vi "Dycometal CCK-25.vi"() -> ()   [LabVIEW 2017]
uses:
  <vilib>/Utility/file.llb/Write Delimited Spreadsheet (DBL).vi
panel:
  out "Frecuencia Fijada":i32=20
  out "Out 1.1":refnum<visa-resource-name>
  out "Out 1.2":errorcluster
  out "Out 2.1":refnum<visa-resource-name>
  out "Out 2.2":errorcluster
  out "Tab Control":enum32{"Comunicación", "Parámetros", "Medición"}(tab)
  in  "Parámetros 1":bool
  in  "Configuración COM - C. Climática":T1={"Velocidad de transmisión"=9600, "Paridad"=0, "Bits de parada"=10} caption="Configuración COM" {"Bits de parada" items=["0"=10, "1,5"=15, "2"=20]; "Paridad" items=["No", "Impar", "Par", "Marcada", "Espaciada"]; "Velocidad de transmisión" items=["300"=300, "600"=600, "1200"=1200, "2400"=2400, "4800"=4800, "9600"=9600]}
  in  "Parámetro prioritario:":bool=TRUE
  in  "Puerto COM - C. Climática":refnum<visa-resource-name> caption="Puerto COM"
  in  "Puerto COM - Medidor LCR":refnum<visa-resource-name> caption="Puerto COM"
  in  "Configuración COM - Medidor LCR":T2={"Velocidad de transmisión"=9600, "Paridad"=0, "Bits de datos"=7, "Bits de parada"=10, "Control flujo de datos"=0} caption="Configuración COM" {"Bits de parada" items=["1"=10, "1,5"=15, "2"=20]; "Bits de datos" items=["7"=7, "8"=8]; "Paridad" items=["No", "Impar", "Par", "Marcada", "Espaciada"]; "Control flujo de datos" items=["No", "XON/XOFF", "RTS/CTS", "XON/XOFF & RTS/CTS", "DTR/DSR", "XON/XOFF & DTR/DSR"]; "Velocidad de transmisión" items=["300"=300, "600"=600, "1200"=1200, "2400"=2400, "4800"=4800, "9600"=9600]}
  in  "Medición 1":bool
  in  "Frecuencia Final":i32(ring)=68 items=["20 Hz", "24 Hz", "25 Hz", "30 Hz", "36 Hz", "40 Hz", "45 Hz", "50 Hz", "60 Hz", "72 Hz", "75 Hz", "80 Hz", "90 Hz", "100 Hz", "120 Hz", "150 Hz", "180 Hz", "200 Hz", "240 Hz", "250 Hz", "300 Hz", "360 Hz", "400 Hz", "450 Hz", "500 Hz", "600 Hz", "720 Hz", "750 Hz", "800 Hz", "900 Hz", "1k Hz", "1,2k Hz", "1,5k Hz", "1,8k Hz", "2k Hz", "2,4k Hz", "2,5k Hz", "3k Hz", "3,6k Hz", "4k Hz", "4,5k Hz", "5k Hz", "6k Hz", "7,2k Hz", "7,5k Hz", "8k Hz", "9k Hz", "10k Hz", "12k Hz", "15k Hz", "18k Hz", "20k Hz", "24k Hz", "25k Hz", "30k Hz", "36k Hz", "40k Hz", "45k Hz", "50k Hz", "60k Hz", "72k Hz", "75k Hz", "80k Hz", "90k Hz", "100k Hz", "120k Hz", "150k Hz", "180k Hz", "200k Hz"]
  in  "Tipo de Circuito":u16(ring)=2 items=["Serie", "Paralelo", "Auto"]
  in  "Formato de Salida":u16(ring) items=["Auto", "L+Q", "L+R", "C+D", "C+R", "R+Q", "Z+Theta", "Y+Theta", "R+X", "G+B", "N+Theta", "M"]
  in  "Escala Manual":u8(ring)=1 items=["Escala 1: 3 Ohms"=1, "Escala 2: 100 Ohms"=2, "Escala 3: 1,6 kOhms"=3, "Escala 4: 25 kOhms"=4, "Escala 5: 500 kOhms"=5, "Escala 6: 100 MOhms"=6]
  in  "Modo Autoescala":bool=TRUE
  in  "Frecuencia Inicial":i32(ring) items=["20 Hz", "24 Hz", "25 Hz", "30 Hz", "36 Hz", "40 Hz", "45 Hz", "50 Hz", "60 Hz", "72 Hz", "75 Hz", "80 Hz", "90 Hz", "100 Hz", "120 Hz", "150 Hz", "180 Hz", "200 Hz", "240 Hz", "250 Hz", "300 Hz", "360 Hz", "400 Hz", "450 Hz", "500 Hz", "600 Hz", "720 Hz", "750 Hz", "800 Hz", "900 Hz", "1k Hz", "1,2k Hz", "1,5k Hz", "1,8k Hz", "2k Hz", "2,4k Hz", "2,5k Hz", "3k Hz", "3,6k Hz", "4k Hz", "4,5k Hz", "5k Hz", "6k Hz", "7,2k Hz", "7,5k Hz", "8k Hz", "9k Hz", "10k Hz", "12k Hz", "15k Hz", "18k Hz", "20k Hz", "24k Hz", "25k Hz", "30k Hz", "36k Hz", "40k Hz", "45k Hz", "50k Hz", "60k Hz", "72k Hz", "75k Hz", "80k Hz", "90k Hz", "100k Hz", "120k Hz", "150k Hz", "180k Hz", "200k Hz"]
  in  "Bol_Escalado_Hum":bool=TRUE
  in  "Bol_Escalado_Temp":bool=TRUE
  in  "Escalado Temp":sgl caption="Escalado" min=0 max=100 step=5
  in  "Error Temp":sgl caption="Error" min=0 max=100
  in  "Error Hum":sgl caption="Error" min=0 max=100
  in  "Escalado Hum":sgl caption="Escalado" min=0 max=100 step=5
  in  "Hum Final":sgl=10.0 caption="Final" min=10 max=98 step=5
  in  "Temp Final":sgl caption="Final" min=0 max=100 step=5
  in  "Temperatura Inicial":sgl caption="Inicio" min=0 max=100 step=5
  in  "Humedad Inicial":sgl=10.0 caption="Inicio" min=10 max=98 step=5
  in  "Ruta a excel de almacenaje":path
  in  "Regimen Permanente":dbl min=0.0 step=900.0 format="%<%H:%M>t"
  in  "Iniciar":bool
  in  "Parámetros 2":bool
  out "Gráfica":T3(graph)={"Temperatura Medida"=20.209763, "Humedad Medida"=41.667168}
  out "Humedad Fijada":sgl
  out "Temperatura Fijada":sgl
  out "En regimen permanente:":dbl format="%<%H:%M>t"
  in  "Obtener datos de gráfica":bool
  out "Últimas mediciones":dbl[][](array[numeric]) format="%^#_4e"
  in  "Parar":bool
  # "Cámara Climática"
  # "Medidor LCR"
  # "Cámara Climática"
  # "Medidor LCR"
  # "¿Bucle en Temperatura o Humedad?"
  # "Última Medición"
  # "Temperatura"
  # "Humedad"
  # "Frecuencia"
  # "Parámetro 1"
  # "Parámetro 2"
  # "Temperatura Medida"
  # "Humedad Medida"
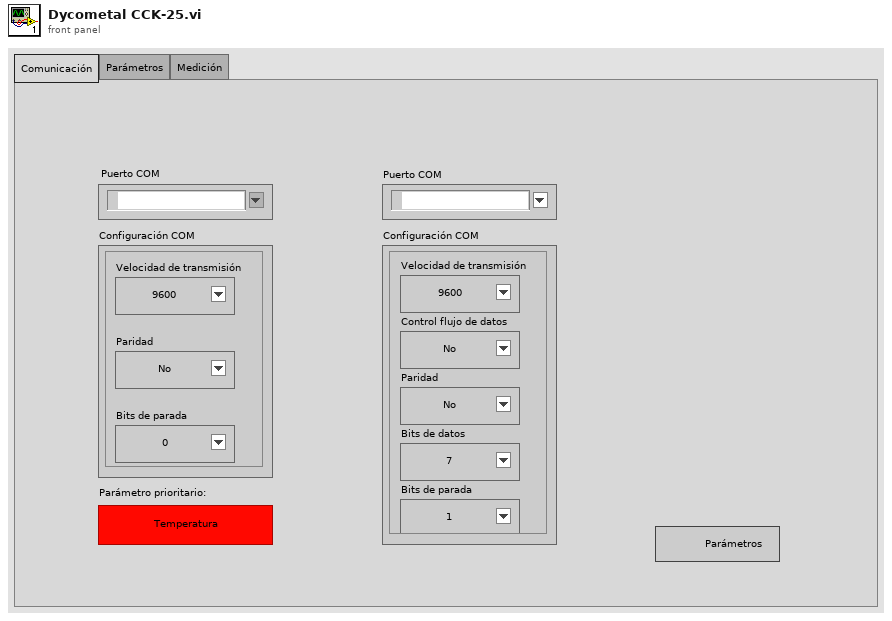
[diagram p1: front panel]
types:
  T1 = cluster{"Velocidad de transmisión":u32, "Paridad":u16, "Bits de parada":u16}
  T2 = cluster{"Velocidad de transmisión":u32, "Paridad":u16, "Bits de datos":u16, "Bits de parada":u16, "Control flujo de datos":u16}
  T3 = cluster{"Temperatura Medida":sgl, "Humedad Medida":sgl}
  T4 = enum8{"Enabled", "Disabled", "Disabled and Grayed Out"}
  T5 = cluster{"Temperatura Medida":sgl, "Humedad Medida":sgl}[]
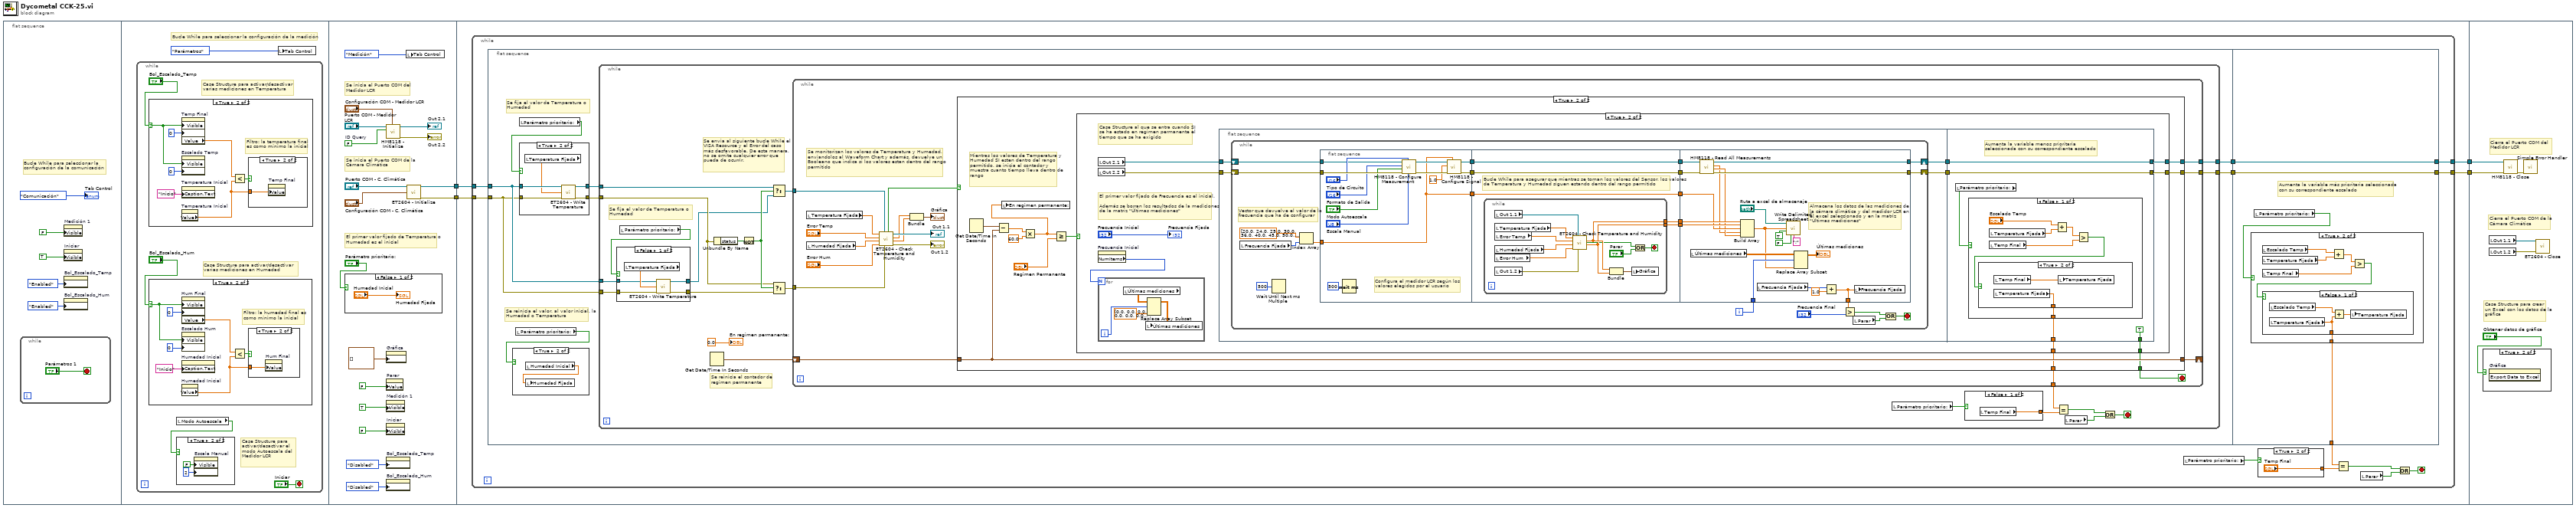
[diagram p0: block diagram]
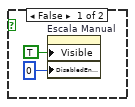
[diagram p2: hidden frame]
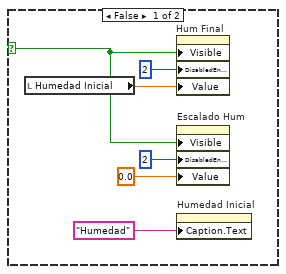
[diagram p3: hidden frame]
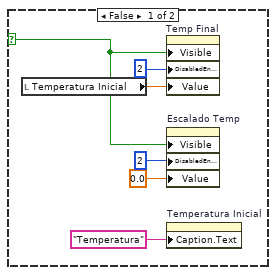
[diagram p5: hidden frame]
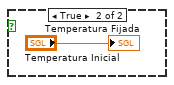
[diagram p7: hidden frame]
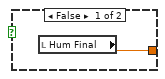
[diagram p8: hidden frame]
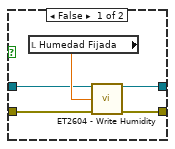
[diagram p9: hidden frame]
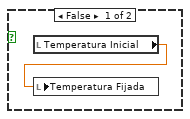
[diagram p10: hidden frame]
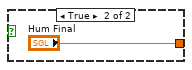
[diagram p11: hidden frame]
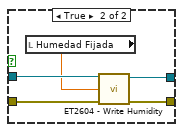
[diagram p12: hidden frame]
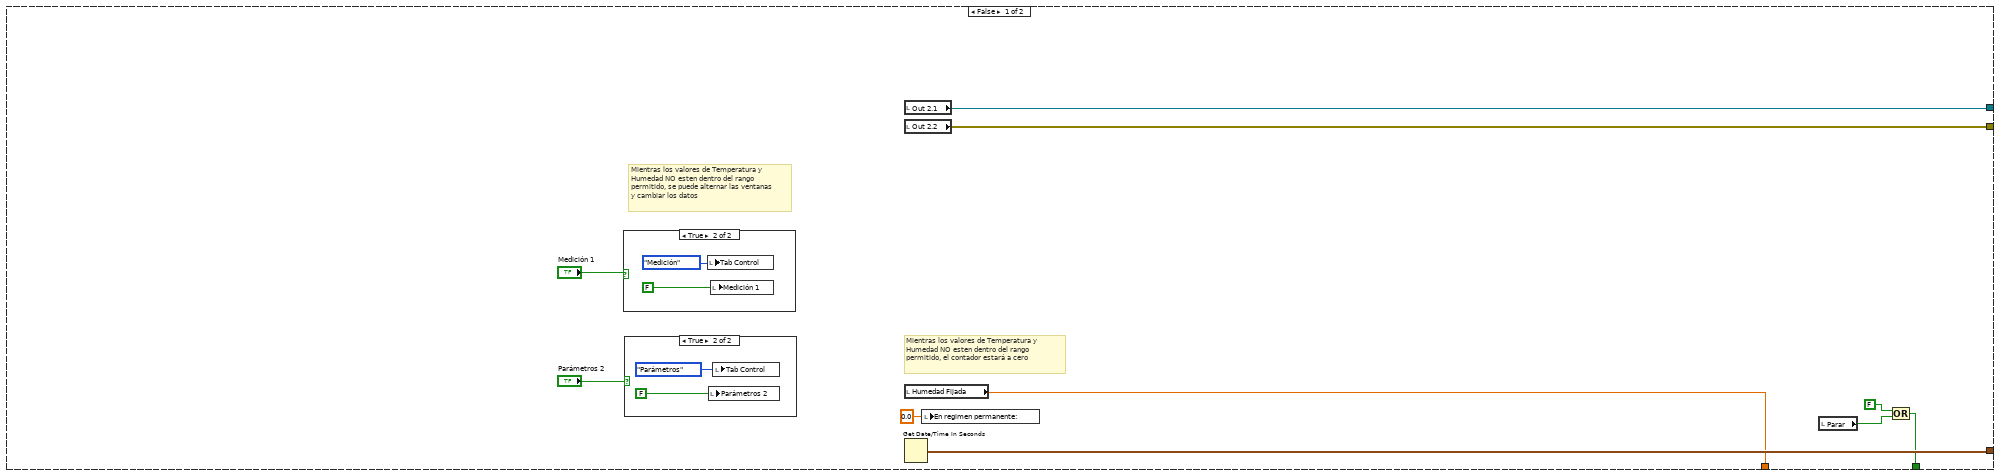
[diagram p13: hidden frame]
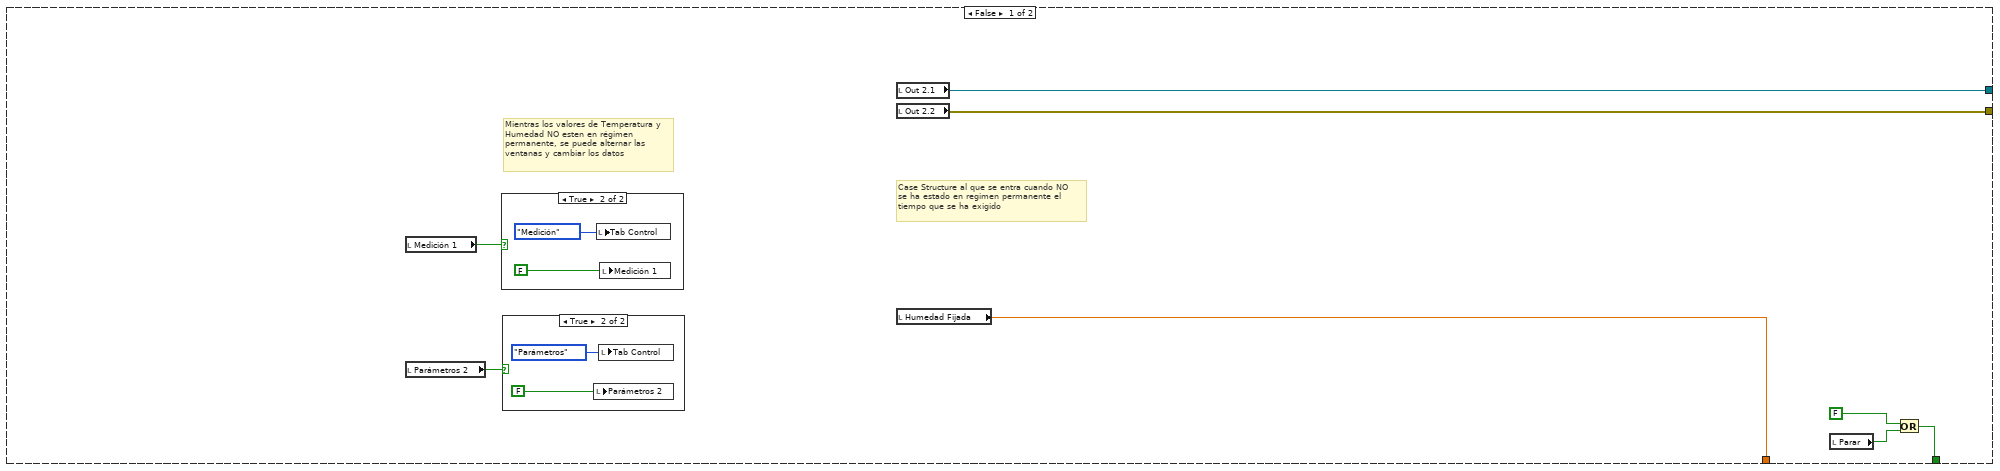
[diagram p16: hidden frame]
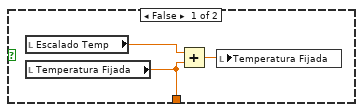
[diagram p19: hidden frame]
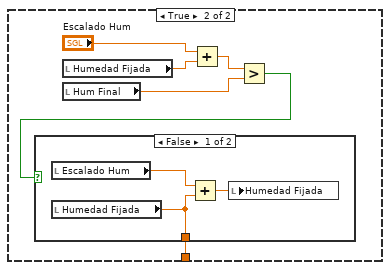
[diagram p20: hidden frame]
diagram:
  n1 = flat-sequence {
    tunnel: [w51] -> w4
    tunnel: [w50] -> w3
    tunnel: w4 -> [w68]
    tunnel: w3 -> [w67]
    tunnel: [w70] -> w2
    tunnel: [w69] -> w1
    tunnel: w2 -> [w339]
    tunnel: w1 -> [w340]
    frame #0 {
      # "Bucle While para seleccionar la configuración de la comunicación"
      n2 = while {
        stop <- "Parámetros 1" stop-if-true
      }
      n3 = property on="Medición 1" class="Bool (strict)"("Visible"=FALSE) -> ()  [unwired: 2 in, 2 out]
      n4 = property on="Iniciar" class="Bool"("Visible"=TRUE) -> ()  [unwired: 2 in, 2 out]
      n5 = property on="Bol_Escalado_Temp" class="Bool (strict)"("DisabledEnum"=T4."Enabled" ("Disabled")) -> ()  [unwired: 2 in, 2 out]
      n6 = property on="Bol_Escalado_Hum" class="Bool (strict)"("DisabledEnum"=T4."Enabled" ("Disabled")) -> ()  [unwired: 2 in, 2 out]
      "Tab Control" <- enum32{"Comunicación", "Parámetros", "Medición"}."Comunicación" ("Tab Control")
    }
    frame #1 {
      # "Bucle While para seleccionar la configuración de la medición"
      n7 = while {
        stop <- "Iniciar" stop-if-true
        # "Case Structure para activar/desactivar el modo Autoescala del Medidor LCR"
        # "Case Structure para activar/desactivar varias mediciones en Humedad"
        # "Case Structure para activar/desactivar varias mediciones en Temperatura"
        n8 = case shown="True" "Bol_Escalado_Temp" {
          selector: "Bol_Escalado_Temp" -> [w39 w46]
          frame False {
            n9 = local read "Temperatura Inicial"() -> (w35:sgl)
            n10 = property on="Temp Final" class="DigNum (strict)"("Visible"=w39, "DisabledEnum"=u8 2, "Value"=w35) -> ()  [unwired: 2 in, 2 out]
            n11 = property on="Escalado Temp" class="DigNum (strict)"("Visible"=w39, "DisabledEnum"=u8 2, "Value"=sgl 0.0 ("Humedad Escalado")) -> ()  [unwired: 2 in, 2 out]
            n12 = property on="Temperatura Inicial" class="DigNum (strict)"("Caption.Text"="Temperatura") -> ()  [unwired: 2 in, 2 out]
          }
          frame True {
            # "Filtro: la temperatura final es como mínimo la inicial"
            n13 = property on="Temp Final" class="DigNum (strict)"("Visible"=w46, "DisabledEnum"=u8 0) -> ("Value"=w42:sgl)  [unwired: 2 in, 2 out]
            n14 = property on="Escalado Temp" class="DigNum (strict)"("Visible"=w46, "DisabledEnum"=u8 0) -> ()  [unwired: 2 in, 2 out]
            n15 = property on="Temperatura Inicial" class="DigNum (strict)"("Caption.Text"="Inicio") -> ()  [unwired: 2 in, 2 out]
            n16 = property on="Temperatura Inicial" class="DigNum (strict)"() -> ("Value"=w40:sgl)  [unwired: 2 in, 2 out]
            n17 = Less?(x=w42, y=w40) -> (x < y?=w41:bool)
            n18 = case shown="True" w41 {
              tunnel: w40 -> [_ w47]
              frame False {
              }
              frame True {
                n19 = property on="Temp Final" class="DigNum (strict)"("Value"=w47) -> ()  [unwired: 2 in, 2 out]
              }
            }
          }
        }
        n20 = case shown="True" "Bol_Escalado_Hum" {
          selector: "Bol_Escalado_Hum" -> [w25 w32]
          frame False {
            n21 = local read "Humedad Inicial"() -> (w21:sgl)
            n22 = property on="Hum Final" class="DigNum (strict)"("Visible"=w25, "DisabledEnum"=u8 2, "Value"=w21) -> ()  [unwired: 2 in, 2 out]
            n23 = property on="Escalado Hum" class="DigNum (strict)"("Visible"=w25, "DisabledEnum"=u8 2, "Value"=sgl 0.0 ("Humedad Escalado")) -> ()  [unwired: 2 in, 2 out]
            n24 = property on="Humedad Inicial" class="DigNum (strict)"("Caption.Text"="Humedad") -> ()  [unwired: 2 in, 2 out]
          }
          frame True {
            # "Filtro: la humedad final es como mínimo la inicial"
            n25 = property on="Hum Final" class="DigNum (strict)"("Visible"=w32, "DisabledEnum"=u8 0) -> ("Value"=w28:sgl)  [unwired: 2 in, 2 out]
            n26 = property on="Escalado Hum" class="DigNum (strict)"("Visible"=w32, "DisabledEnum"=u8 0) -> ()  [unwired: 2 in, 2 out]
            n27 = property on="Humedad Inicial" class="DigNum (strict)"("Caption.Text"="Inicio") -> ()  [unwired: 2 in, 2 out]
            n28 = property on="Humedad Inicial" class="DigNum (strict)"() -> ("Value"=w27:sgl)  [unwired: 2 in, 2 out]
            n29 = Less?(x=w28, y=w27) -> (x < y?=w26:bool)
            n30 = case shown="True" w26 {
              tunnel: w27 -> [_ w33]
              frame False {
              }
              frame True {
                n31 = property on="Hum Final" class="DigNum (strict)"("Value"=w33) -> ()  [unwired: 2 in, 2 out]
              }
            }
          }
        }
        n32 = local read "Modo Autoescala"() -> (w12:bool)
        n33 = case shown="True" w12 {
          frame False {
            n34 = property on="Escala Manual" class="Ring (strict)"("Visible"=TRUE, "DisabledEnum"=u8 0) -> ()  [unwired: 2 in, 2 out]
          }
          frame True {
            n35 = property on="Escala Manual" class="Ring (strict)"("Visible"=FALSE, "DisabledEnum"=u8 2) -> ()  [unwired: 2 in, 2 out]
          }
        }
      }
      n36 = local write "Tab Control"(enum32{"Comunicación", "Parámetros", "Medición"}."Parámetros" ("Tab Control")) -> ()
    }
    frame #2 {
      w52 = FALSE  # ID Query
      # "El primer valor fijado de Temperatura o Humedad es el inicial"
      # "Se inicia el Puerto COM de la Cámara Climática"
      # "Se inicia el Puerto COM del Medidor LCR"
      n37 = case shown="False" "Parámetro prioritario:" {
        frame False {
          "Humedad Fijada" <- "Humedad Inicial"
        }
        frame True {
          "Temperatura Fijada" <- "Temperatura Inicial"
        }
      }
      n38 = call "HM8118 - Initialize.vi"("Serial Configuration"="Configuración COM - Medidor LCR", "ID Query (True)"=w52, "VISA resource name"="Puerto COM - Medidor LCR") -> ("error out"=→"Out 2.2":errorcluster, "VISA resource name out"=→"Out 2.1":refnum<visa-resource-name>)  [unwired: 7 in]
      n39 = property on="Gráfica" class="WFChart (strict)"("History Data"=T5 []) -> ()  [unwired: 2 in, 2 out]
      n40 = property on="Parar" class="Bool (strict)"("Value"=FALSE ("Cancel Button")) -> ()  [unwired: 2 in, 2 out]
      n41 = property on="Medición 1" class="Bool (strict)"("Visible"=TRUE) -> ()  [unwired: 2 in, 2 out]
      n42 = property on="Iniciar" class="Bool"("Visible"=FALSE) -> ()  [unwired: 2 in, 2 out]
      n43 = property on="Bol_Escalado_Temp" class="Bool (strict)"("DisabledEnum"=T4."Disabled" ("Disabled")) -> ()  [unwired: 2 in, 2 out]
      n44 = property on="Bol_Escalado_Hum" class="Bool (strict)"("DisabledEnum"=T4."Disabled" ("Disabled")) -> ()  [unwired: 2 in, 2 out]
      n45 = local write "Tab Control"(enum32{"Comunicación", "Parámetros", "Medición"}."Medición" ("Tab Control")) -> ()
      n46 = call "ET2604 - Initialize.vi"("VISA resource name"="Puerto COM - C. Climática", "Serial Configuration"="Configuración COM - C. Climática") -> ("VISA resource name out"=w51:refnum<visa-resource-name>, "error out"=w50:errorcluster)  [unwired: 12 in]
    }
    frame #3 {
      n47 = while {
        tunnel: w67 -> [w79]
        tunnel: [w81] -> w69
        tunnel: w68 -> [w80]
        tunnel: [w82] -> w70
        stop <- w72 stop-if-true
        n48 = flat-sequence {
          tunnel: w80 -> [w86]
          tunnel: w79 -> [w85]
          tunnel: [w90] -> w78
          tunnel: [w89] -> w77
          tunnel: [w312] -> w81
          tunnel: [w313] -> w82
          tunnel: w78 -> [w313]
          tunnel: w77 -> [w312]
          tunnel: [w311] -> w75
          frame #0 {
            # "Se reinicia el valor, al valor inicial, la Humedad o Temperatura"
            # "Se fija el valor de Temperatura o Humedad"
            n49 = local read "Parámetro prioritario:"() -> (w88:bool)
            n50 = case shown="True" w88 {
              frame False {
                n51 = local read "Temperatura Inicial"() -> (w103:sgl)
                n52 = local write "Temperatura Fijada"(w103) -> ()
              }
              frame True {
                n53 = local read "Humedad Inicial"() -> (w104:sgl)
                n54 = local write "Humedad Fijada"(w104) -> ()
              }
            }
            n55 = local read "Parámetro prioritario:"() -> (w87:bool)
            n56 = case shown="True" w87 {
              tunnel: [w97 w101] -> w92
              tunnel: [w96 w102] -> w91
              tunnel: w86 -> [w93 w100]
              tunnel: w85 -> [w95 w99]
              frame False {
                n57 = local read "Humedad Fijada"() -> (w94:sgl)
                n58 = call "ET2604 - Write Humidity.vi"("VISA resource name"=w93, "Data (0)"=w94, "error in (no error)"=w95) -> ("VISA resource name out"=w97:refnum<visa-resource-name>, "error out"=w96:errorcluster)  [unwired: 11 in]
              }
              frame True {
                n59 = local read "Temperatura Fijada"() -> (w98:sgl)
                n60 = call "ET2604 - Write Temperature.vi"("VISA resource name"=w100, "Data (0)"=w98, "error in (no error)"=w99) -> ("VISA resource name out"=w101:refnum<visa-resource-name>, "error out"=w102:errorcluster)  [unwired: 11 in]
              }
            }
            n61 = while {
              tunnel: w86 -> [w123]
              tunnel: w85 -> [w122]
              tunnel: w92 -> [w108]
              tunnel: [w125] -> w90
              tunnel: w91 -> [w107]
              tunnel: [w124] -> w89
              stop <- w116 stop-if-true
              # "Se reinicia el contador de regimen permanente"
              # "Se envia al siguiente bucle While el VISA Resource y el Error del caso más desfavorable. De esta manera, no se omite cualquier error que pueda de ocurrir."
              # "Se fija el valor de Temperatura o Humedad"
              n62 = local read "Parámetro prioritario:"() -> (w118:bool)
              n63 = case shown="False" w118 {
                tunnel: [w132 w137] -> w106
                tunnel: [w131 w136] -> w112
                tunnel: w123 -> [w128 w134]
                tunnel: w122 -> [w130 w135]
                frame False {
                  n64 = local read "Temperatura Fijada"() -> (w129:sgl)
                  n65 = call "ET2604 - Write Temperature.vi"("VISA resource name"=w128, "Data (0)"=w129, "error in (no error)"=w130) -> ("VISA resource name out"=w132:refnum<visa-resource-name>, "error out"=w131:errorcluster)  [unwired: 11 in]
                }
                frame True {
                  n66 = local read "Humedad Fijada"() -> (w133:sgl)
                  n67 = call "ET2604 - Write Humidity.vi"("VISA resource name"=w134, "Data (0)"=w133, "error in (no error)"=w135) -> ("VISA resource name out"=w137:refnum<visa-resource-name>, "error out"=w136:errorcluster)  [unwired: 11 in]
                }
              }
              n68 = Get Date/Time In Seconds() -> (seconds since 1Jan1904=w119:timestamp)
              n69 = Unbundle By Name(w107) -> ("status"=w113:bool)
              n70 = Not(x=w113) -> (.not. x?=w111:bool)
              n71 = Select(t=w108, s=w111, f=w106) -> (s? t:f=w110:refnum<visa-resource-name>)
              n72 = Select(t=w107, s=w111, f=w112) -> (s? t:f=w109:errorcluster)
              n73 = while {
                shift-right: [w155] -> _
                shift-left: w119 -> [w154]
                tunnel: [w153] -> w125
                tunnel: [w152] -> w124
                tunnel: [w151] -> w120
                tunnel: w110 -> [w142]
                tunnel: w109 -> [w146]
                stop <- w150 stop-if-true
                # "Se monitorizan los valores de Temperatura y Humedad, enviandolos al Waveform Chart y además, devuelve un Booleano que indica si los valores estan dentro del rango permitido"
                n74 = local read "Temperatura Fijada"() -> (w141:sgl)
                n75 = local read "Humedad Fijada"() -> (w139:sgl)
                n76 = call "ET2604 - Check Temperature and Humidity.vi"("error in (no error)"=w146, "VISA input"=w142, "Error de Humedad"="Error Hum", "Humedad Fijada"=w139, "Error de Temperatura"="Error Temp", "Temperatura Fijada"=w141) -> ("error out"=→"Out 1.2":errorcluster, "Humedad Medida"=w145:sgl, "Temperatura Medida"=w144:sgl, "VISA output"=→"Out 1.1":refnum<visa-resource-name>, "¿En Rango?"=w143:bool)
                n77 = Bundle("Temperatura Medida"=w144, "Humedad Medida"=w145) -> (→"Gráfica":T3)  [unwired: 1 in]
                n78 = case shown="True" w143 {
                  tunnel: [w165 w178] -> w155
                  tunnel: w154 -> [_ w178]
                  tunnel: [w163 w176] -> w153
                  tunnel: [w162 w175] -> w152
                  tunnel: [w161 w174] -> w151
                  tunnel: [w160 w173] -> w150
                  frame False {
                    # "Mientras los valores de Temperatura y Humedad NO esten dentro del rango permitido, se puede alternar las ventanas y cambiar los datos"
                    # "Mientras los valores de Temperatura y Humedad NO esten dentro del rango permitido, el contador estará a cero"
                    n79 = case shown="True" "Medición 1" {
                      frame False {
                      }
                      frame True {
                        n80 = local write "Tab Control"(enum32{"Comunicación", "Parámetros", "Medición"}."Medición" ("Tab Control")) -> ()
                        n81 = local write "Medición 1"(FALSE ("Medición 1")) -> ()
                      }
                    }
                    n82 = case shown="True" "Parámetros 2" {
                      frame False {
                      }
                      frame True {
                        n83 = local write "Parámetros 2"(FALSE ("Parámetros 2")) -> ()
                        n84 = local write "Tab Control"(enum32{"Comunicación", "Parámetros", "Medición"}."Parámetros" ("Tab Control")) -> ()
                      }
                    }
                    n85 = local read "Out 2.1"() -> (w163:refnum<visa-resource-name>)
                    n86 = local read "Out 2.2"() -> (w162:errorcluster)
                    n87 = local read "Humedad Fijada"() -> (w161:sgl)
                    n88 = Get Date/Time In Seconds() -> (seconds since 1Jan1904=w165:timestamp)
                    n89 = local write "En regimen permanente:"(0.0 ("Tiempo Transcurrido")) -> ()
                    n90 = local read "Parar"() -> (w158:bool)
                    n91 = Or(x=FALSE, y=w158) -> (x .or. y?=w160:bool)
                  }
                  frame True {
                    # "Mientras los valores de Temperatura y Humedad SI esten dentro del rango permitido, se inicia el contador y muestra cuanto tiempo lleva dentro de rango"
                    n92 = Get Date/Time In Seconds() -> (seconds since 1Jan1904=w180:timestamp)
                    n93 = Subtract(x=w180, y=w178) -> (x-y=w171:dbl)
                    n94 = Multiply(x=w171, y=60.0) -> (x*y=w170:dbl)
                    n95 = local write "En regimen permanente:"(w170) -> ()
                    n96 = Greater Or Equal?(x=w170, y="Regimen Permanente") -> (x >= y?=w177:bool)
                    n97 = case shown="True" w177 {
                      tunnel: [w188 w201] -> w176
                      tunnel: [w187 w200] -> w175
                      tunnel: [w186 w196] -> w174
                      tunnel: [w185 w195] -> w173
                      frame False {
                        # "Mientras los valores de Temperatura y Humedad NO esten en régimen permanente, se puede alternar las ventanas y cambiar los datos"
                        # "Case Structure al que se entra cuando NO se ha estado en regimen permanente el tiempo que se ha exigido"
                        n98 = local read "Medición 1"() -> (w182:bool)
                        n99 = local read "Parámetros 2"() -> (w181:bool)
                        n100 = case shown="True" w182 {
                          frame False {
                          }
                          frame True {
                            n101 = local write "Tab Control"(enum32{"Comunicación", "Parámetros", "Medición"}."Medición" ("Tab Control")) -> ()
                            n102 = local write "Medición 1"(FALSE ("Medición 1")) -> ()
                          }
                        }
                        n103 = case shown="True" w181 {
                          frame False {
                          }
                          frame True {
                            n104 = local write "Parámetros 2"(FALSE ("Parámetros 2")) -> ()
                            n105 = local write "Tab Control"(enum32{"Comunicación", "Parámetros", "Medición"}."Parámetros" ("Tab Control")) -> ()
                          }
                        }
                        n106 = local read "Out 2.1"() -> (w188:refnum<visa-resource-name>)
                        n107 = local read "Out 2.2"() -> (w187:errorcluster)
                        n108 = local read "Humedad Fijada"() -> (w186:sgl)
                        n109 = local read "Parar"() -> (w183:bool)
                        n110 = Or(x=FALSE, y=w183) -> (x .or. y?=w185:bool)
                      }
                      frame True {
                        # "Case Structure al que se entra cuando SI se ha estado en regimen permanente el tiempo que se ha exigido"
                        # "El primer valor fijado de Frecuencia es el inicial.\n\nAdemás se borran los resultados de la mediciones de la matriz \"Últimas mediciones\""
                        n111 = local read "Out 2.1"() -> (w202:refnum<visa-resource-name>)
                        n112 = local read "Out 2.2"() -> (w194:errorcluster)
                        n113 = property on="Frecuencia Inicial" class="Ring (strict)"() -> ("NumItems"=w193:u32)  [unwired: 2 in, 2 out]
                        n114 = for {
                          N: w193 -> [_]
                          i -> [w205]
                          n115 = local read "Últimas mediciones"() -> (w206:dbl[][])
                          n116 = Replace Array Subset(array=w206, new element=dbl[] [0.0, 0.0, 0.0, 0.0, 0.0, 0.0, 0.0, 0.0, 0.0, 0.0, 0.0, 0.0, 0.0, 0.0, 0.0, 0.0, 0.0, 0.0, 0.0, 0.0, 0.0, 0.0, 0.0, 0.0, 0.0, 0.0, 0.0, 0.0, 0.0, 0.0, 0.0, 0.0, 0.0, 0.0, 0.0, 0.0, 0.0, 0.0, 0.0, 0.0, 0.0, 0.0, 0.0, 0.0, 0.0, 0.0, 0.0, 0.0, 0.0, 0.0, 0.0, 0.0, 0.0, 0.0, 0.0, 0.0, 0.0, 0.0, 0.0, 0.0, 0.0, 0.0, 0.0, 0.0, 0.0, 0.0, 0.0, 0.0, 0.0] ("new element/subarray"), index (row)=w205) -> (w203:dbl[][])  [unwired: 1 in]
                          n117 = local write "Últimas mediciones"(w203) -> ()
                        }
                        n118 = flat-sequence {
                          tunnel: w202 -> [w210]
                          tunnel: w194 -> [w209]
                          tunnel: [w208] -> w198
                          tunnel: [w207] -> w197
                          tunnel: [w286] -> w200
                          tunnel: [w287] -> w201
                          tunnel: w198 -> [w287]
                          tunnel: w197 -> [w286]
                          tunnel: [w285] -> w196
                          tunnel: [TRUE] -> w195
                          frame #0 {
                            n119 = while {
                              shift-right: [w227] -> w208
                              shift-left: w210 -> [w231]
                              shift-right: [w228] -> w207
                              shift-left: w209 -> [w230]
                              i -> [w212]
                              stop <- w217 stop-if-true
                              # "Vector que devuelve el valor de la frecuencia que ha de configurar"
                              n120 = local read "Frecuencia Fijada"() -> (w219:i32)
                              n121 = Wait Until Next ms Multiple(millisecond multiple=u32 500) -> ()  [unwired: 1 out]
                              n122 = Index Array(array=dbl[] [20.0, 24.0, 25.0, 30.0, 36.0, 40.0, 45.0, 50.0, 60.0, 72.0, 75.0, 80.0, 90.0, 100.0, 120.0, 150.0, 180.0, 200.0, 240.0, 250.0, 300.0, 360.0, 400.0, 450.0, 500.0, 600.0, 720.0, 750.0, 800.0, 900.0, 1000.0, 1200.0, 1500.0, 1800.0, 2000.0, 2400.0, 2500.0, 3000.0, 3600.0, 4000.0, 4500.0, 5000.0, 6000.0, 7200.0, 7500.0, 8000.0, 9000.0, 10000.0, 12000.0, 15000.0, 18000.0, 20000.0, 24000.0, 25000.0, 30000.0, 36000.0, 40000.0, 45000.0, 50000.0, 60000.0, 72000.0, 75000.0, 80000.0, 90000.0, 100000.0, 120000.0, 150000.0, 180000.0, 200000.0], index=w219) -> (element=w222:dbl)
                              n123 = flat-sequence {
                                tunnel: w231 -> [w239]
                                tunnel: w230 -> [w244]
                                tunnel: [w238] -> w229
                                tunnel: w222 -> [w234]
                                tunnel: [w234] -> w214
                                tunnel: [w237] -> w211
                                tunnel: w229 -> [w249]
                                tunnel: [w249] -> w224
                                tunnel: [w250] -> w223
                                tunnel: [w248] -> w221
                                tunnel: [w247] -> w220
                                tunnel: w214 -> [w246]
                                tunnel: [w246] -> w213
                                tunnel: w211 -> [w250]
                                tunnel: [w271] -> w227
                                tunnel: [w270] -> w228
                                tunnel: w224 -> [w273]
                                tunnel: w223 -> [w272]
                                tunnel: w221 -> [w279]
                                tunnel: w220 -> [w278]
                                tunnel: [w280] -> w218
                                tunnel: w212 -> [w275]
                                tunnel: w213 -> [w274]
                                frame #0 {
                                # "Configura el medidor LCR según los valores elegidos por el usuario"
                                n124 = Wait (ms)(milliseconds to wait=u32 500) -> ()  [unwired: 1 out]
                                n125 = call "HM8118 - Configure Measurement.vi"("Manual Range (1:Range 1 and 25 Ohms)"="Escala Manual", "Circuit Type (2: Auto)"="Tipo de Circuito", "error in (no error)"=w244, "Auto Range (T: Enable)"="Modo Autoescala", "Operation Mode (0: Auto)"="Formato de Salida", "VISA resource name"=w239) -> ("error out"=w235:errorcluster, "VISA resource name out"=w236:refnum<visa-resource-name>)  [unwired: 4 in]
                                n126 = call "HM8118 - Configure Signal.vi"("Frequency (1kHz)"=w234, "error in (no error)"=w235, "Measuring Voltage (1V)"=1.0, "VISA resource name"=w236) -> ("error out"=w238:errorcluster, "VISA resource name out"=w237:refnum<visa-resource-name>)  [unwired: 6 in]
                                }
                                frame #1 {
                                # "Bucle While para asegurar que mientras se toman los valores del Sensor, los valores de Temperatura y Humedad siguen estando dentro del rango permitido"
                                n127 = while {
                                tunnel: [w253] -> w248
                                tunnel: [w252] -> w247
                                stop <- w261 stop-if-true
                                n128 = local read "Out 1.1"() -> (w254:refnum<visa-resource-name>)
                                n129 = local read "Temperatura Fijada"() -> (w259:sgl)
                                n130 = local read "Error Temp"() -> (w258:sgl)
                                n131 = local read "Humedad Fijada"() -> (w257:sgl)
                                n132 = local read "Error Hum"() -> (w256:sgl)
                                n133 = local read "Out 1.2"() -> (w255:errorcluster)
                                n134 = call "ET2604 - Check Temperature and Humidity.vi"("error in (no error)"=w255, "VISA input"=w254, "Error de Humedad"=w256, "Humedad Fijada"=w257, "Error de Temperatura"=w258, "Temperatura Fijada"=w259) -> ("Humedad Medida"=w252:sgl, "Temperatura Medida"=w253:sgl, "¿En Rango?"=w251:bool)  [unwired: 2 out]
                                n135 = Bundle("Temperatura Medida"=w253, "Humedad Medida"=w252) -> (w262:T3)  [unwired: 1 in]
                                n136 = local write "Gráfica"(w262) -> ()
                                n137 = Or(x=w251, y="Parar") -> (x .or. y?=w261:bool)
                                }
                                }
                                frame #2 {
                                # "Almacena los datos de las mediciones de la cámara climática y del medidor LCR en el excel seleccionado y en la matriz \"Últimas mediciones\""
                                n138 = local read "Últimas mediciones"() -> (w277:dbl[][])
                                n139 = call "HM8118 - Read All Measurements.vi"("error in (no error)"=w273, "VISA resource name"=w272) -> ("error out"=w270:errorcluster, "Secondary"=w269:dbl, "Primary"=w268:dbl, "VISA resource name out"=w271:refnum<visa-resource-name>)  [unwired: 5 in, 1 out]
                                n140 = Build Array(w279, w278, w274, w268, w269) -> (w264:dbl[])
                                n141 = local read "Frecuencia Fijada"() -> (w281:i32)
                                n142 = call-poly <vilib>:"Write Delimited Spreadsheet.vi"("file path (dialog if empty)"="Ruta a excel de almacenaje", "1D data"=w264, "append to file? (new file:F)"=TRUE, "transpose? (no:F)"=FALSE, "delimiter (\\t)"=";" ("delimiter (\\t)")) -> ()  [unwired: 9 in, 2 out]
                                n143 = Replace Array Subset(array=w277, new element=w264, index (row)=w275) -> (→"Últimas mediciones":dbl[][])  [unwired: 1 in]
                                n144 = Add(x=w281, y=1.0) -> (x+y=w280:dbl)
                                n145 = local write "Frecuencia Fijada"(w280) -> ()
                                }
                              }
                              n146 = Greater?(x=w218, y="Frecuencia Final") -> (0:w216:bool)
                              n147 = local read "Parar"() -> (w215:bool)
                              n148 = Or(x=w216, y=w215) -> (x .or. y?=w217:bool)
                            }
                          }
                          frame #1 {
                            # "Aumenta la variable menos prioritaria seleccionada con su correspondiente escalado"
                            n149 = local read "Parámetro prioritario:"() -> (w283:bool)
                            n150 = case shown="False" w283 {
                              tunnel: [w289 w304] -> w285
                              frame False {
                                n151 = local read "Temperatura Fijada"() -> (w293:sgl)
                                n152 = local read "Temp Final"() -> (w291:sgl)
                                n153 = Add(x="Escalado Temp", y=w293) -> (x+y=w292:sgl)
                                n154 = Greater?(x=w292, y=w291) -> (0:w290:bool)
                                n155 = case shown="True" w290 {
                                tunnel: [w294 w297] -> w289
                                frame False {
                                n156 = local read "Escalado Temp"() -> (w296:sgl)
                                n157 = local read "Temperatura Fijada"() -> (w294:sgl)
                                n158 = Add(x=w296, y=w294) -> (x+y=w295:sgl)
                                n159 = local write "Temperatura Fijada"(w295) -> ()
                                }
                                frame True {
                                n160 = local read "Temp Final"() -> (w298:sgl)
                                n161 = local read "Temperatura Fijada"() -> (w297:sgl)
                                n162 = local write "Temperatura Fijada"(w298) -> ()
                                }
                                }
                              }
                              frame True {
                                n163 = local read "Humedad Fijada"() -> (w301:sgl)
                                n164 = local read "Hum Final"() -> (w302:sgl)
                                n165 = Add(x="Escalado Hum", y=w301) -> (x+y=w303:sgl)
                                n166 = Greater?(x=w303, y=w302) -> (0:w299:bool)
                                n167 = case shown="False" w299 {
                                tunnel: [w305 w308] -> w304
                                frame False {
                                n168 = local read "Escalado Hum"() -> (w306:sgl)
                                n169 = local read "Humedad Fijada"() -> (w305:sgl)
                                n170 = Add(x=w306, y=w305) -> (x+y=w307:sgl)
                                n171 = local write "Humedad Fijada"(w307) -> ()
                                }
                                frame True {
                                n172 = local read "Hum Final"() -> (w309:sgl)
                                n173 = local read "Humedad Fijada"() -> (w308:sgl)
                                n174 = local write "Humedad Fijada"(w309) -> ()
                                }
                                }
                              }
                            }
                          }
                        }
                        "Frecuencia Fijada" <- "Frecuencia Inicial"
                      }
                    }
                  }
                }
              }
              n175 = local read "Parámetro prioritario:"() -> (w117:bool)
              n176 = case shown="False" w117 {
                tunnel: [w126 "Hum Final"] -> w121
                frame False {
                  n177 = local read "Temp Final"() -> (w126:sgl)
                }
                frame True {
                }
              }
              n178 = Equal?(x=w120, y=w121) -> (x = y?=w115:bool)
              n179 = local read "Parar"() -> (w114:bool)
              n180 = Or(x=w115, y=w114) -> (x .or. y?=w116:bool)
              "En regimen permanente:" <- 0.0
            }
          }
          frame #1 {
            # "Aumenta la variable más prioritaria seleccionada con su correspondiente escalado"
            n181 = local read "Parámetro prioritario:"() -> (w310:bool)
            n182 = case shown="True" w310 {
              tunnel: [w314 w326] -> w311
              frame False {
                n183 = local read "Escalado Hum"() -> (w319:sgl)
                n184 = local read "Humedad Fijada"() -> (w318:sgl)
                n185 = local read "Hum Final"() -> (w317:sgl)
                n186 = Add(x=w319, y=w318) -> (x+y=w316:sgl)
                n187 = Greater?(x=w316, y=w317) -> (0:w315:bool)
                n188 = case shown="True" w315 {
                  tunnel: [w320 w323] -> w314
                  frame False {
                    n189 = local read "Escalado Hum"() -> (w322:sgl)
                    n190 = local read "Humedad Fijada"() -> (w320:sgl)
                    n191 = Add(x=w322, y=w320) -> (x+y=w321:sgl)
                    n192 = local write "Humedad Fijada"(w321) -> ()
                  }
                  frame True {
                    n193 = local read "Hum Final"() -> (w324:sgl)
                    n194 = local read "Humedad Fijada"() -> (w323:sgl)
                    n195 = local write "Humedad Fijada"(w324) -> ()
                  }
                }
              }
              frame True {
                n196 = local read "Escalado Temp"() -> (w325:sgl)
                n197 = local read "Temperatura Fijada"() -> (w330:sgl)
                n198 = local read "Temp Final"() -> (w329:sgl)
                n199 = Add(x=w325, y=w330) -> (x+y=w328:sgl)
                n200 = Greater?(x=w328, y=w329) -> (0:w327:bool)
                n201 = case shown="False" w327 {
                  tunnel: [w331 w334] -> w326
                  frame False {
                    n202 = local read "Escalado Temp"() -> (w333:sgl)
                    n203 = local read "Temperatura Fijada"() -> (w331:sgl)
                    n204 = Add(x=w333, y=w331) -> (x+y=w332:sgl)
                    n205 = local write "Temperatura Fijada"(w332) -> ()
                  }
                  frame True {
                    n206 = local read "Temp Final"() -> (w335:sgl)
                    n207 = local read "Temperatura Fijada"() -> (w334:sgl)
                    n208 = local write "Temperatura Fijada"(w335) -> ()
                  }
                }
              }
            }
          }
        }
        n209 = local read "Parámetro prioritario:"() -> (w74:bool)
        n210 = case shown="True" w74 {
          tunnel: [w83 "Temp Final"] -> w76
          frame False {
            n211 = local read "Hum Final"() -> (w83:sgl)
          }
          frame True {
          }
        }
        n212 = Equal?(x=w75, y=w76) -> (x = y?=w73:bool)
        n213 = local read "Parar"() -> (w71:bool)
        n214 = Or(x=w73, y=w71) -> (x .or. y?=w72:bool)
      }
    }
    frame #4 {
      # "Case Structure para crear un Excel con los datos de la gráfica"
      # "Cierra el Puerto COM de la Cámara Climática"
      # "Cierra el Puerto COM del Medidor LCR"
      n215 = case shown="True" "Obtener datos de gráfica" {
        frame False {
        }
        frame True {
          n216 = invoke on="Gráfica" class="WFChart (strict)" method="Export Data to Excel"() -> ()  [unwired: 3 in, 3 out]
        }
      }
      n217 = local read "Out 1.1"() -> (w337:refnum<visa-resource-name>)
      n218 = local read "Out 1.2"() -> (w336:errorcluster)
      n219 = call "HM8118 - Close.vi"("VISA resource name"=w339, "error in (no error)"=w340) -> ("error out"=w338:errorcluster)  [unwired: 8 in]
      n220 = call <vilib>:"Simple Error Handler.vi"("error in (no error)"=w338) -> ()  [unwired: 4 in, 5 out]
      n221 = call "ET2604 - Close.vi"("VISA resource name"=w337, "error in (no error)"=w336) -> ()  [unwired: 13 in, 1 out]
    }
  }
